vi "target.vi"   [LabVIEW 2020]
uses:
  <vilib>/rvi/DataTransferAndStorage/Container/XNode/niFpgaContainer.xnode
  <vilib>/rvi/interface/RandomDataEmulation/nirviRandomDataFpgaReadWriteTemplate.vi
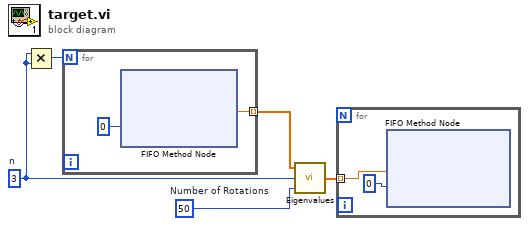
[diagram p0: block diagram]
diagram:
  w2 = 50  # Number of Rotations
  w3 = 3  # n
  n1 = Multiply(x=w3, y=w3) -> (x*y=w5:i32)
  n2 = for {
    N: w5 -> [_]
    tunnel: [w7] -> w4 mode=indexing
    n3 = xnode ("FIFO Method Node")("Timeout"=0) -> ("Element"=w7:sgl)  [unwired: 1 in, 2 out]
  }
  n4 = call "Eigenvalues.vi"("Number of Rotations (100)"=w2, "n"=w3, "A"=w4) -> ("eigenvalues"=w1:sgl[])
  n5 = for {
    tunnel: w1 -> [w8] mode=indexing
    n6 = xnode ("FIFO Method Node")("Element"=w8, "Timeout"=0) -> ()  [unwired: 1 in, 2 out]
  }
